vi "State Machine Kernel.vi"(4 "Init?":bool, 5 "Inputs":T3 {"Kobuki Sensors"."Charger Source" items=["DISCHARGING"=0, "DOCKING_CHARGED"=2, "DOCKING_CHARGING"=6, "ADAPTER_CHARGED"=18, "ADAPTER_CHARGING"=22]; "accelerometer"."z axis (g)" format="%.3f"; "accelerometer"."y axis (g)" format="%.3f"; "accelerometer"."x axis (g)" format="%.3f"}, 7 "StateIn":T1=enum."Init") -> (0 "Terminated?":bool, 2 "Outputs":T2, 3 "StateOut":T1=enum."Init")   [LabVIEW 2017]
uses:
  Statechart.lvsc/Inputs.ctl
  shared/Accelerometer.ctl
  Kobuki/KobukiSensors.ctl
  Kobuki/Kobuki Bumps and WheelDrops.ctl
  Kobuki/Kobuki Buttons.ctl
  Statechart.lvsc/Outputs.ctl
  StatesEnum.ctl
  Statechart.lvsc
panel:
  # "Electrical: charging, battery, OI mode"
  # "Sensors: bump, cliff, button, wheel drop"
  # "Motors:"
  # "Inertia"
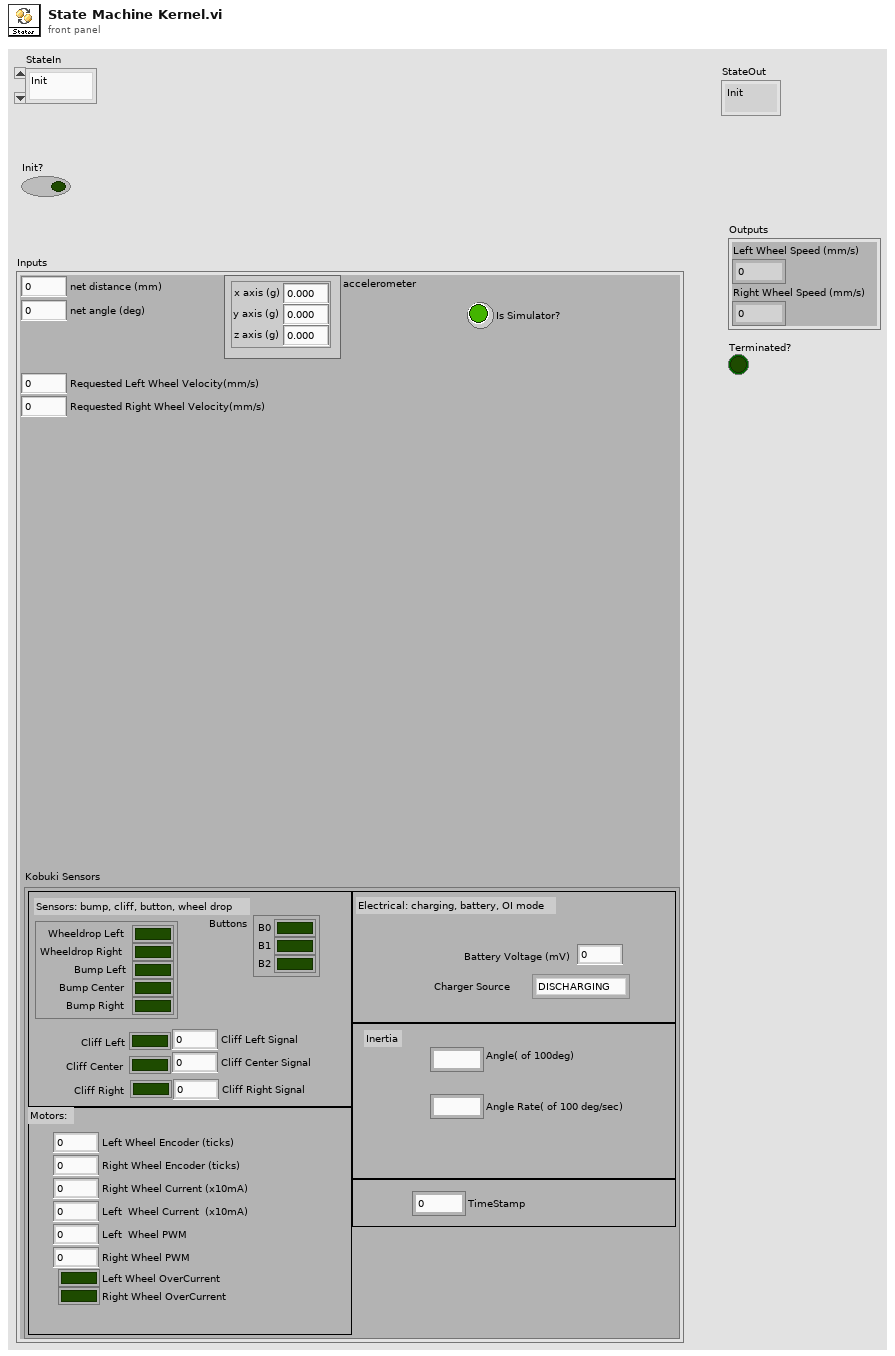
[diagram p1: front panel]
types:
  T1 = typedef "StatesEnum.ctl" = enum16{"Pause", "Init", "Shut"}
  T2 = typedef "Statechart.lvsc/Outputs.ctl" = cluster{"Left Wheel Speed (mm/s)":i16, "Right Wheel Speed (mm/s)":i16}
  T3 = typedef "Statechart.lvsc/Inputs.ctl" = cluster{"net distance (mm)":i32, "net angle (deg)":i32, "accelerometer":T4, "Is Simulator?":bool, "Kobuki Sensors":T5, "Requested Left Wheel Velocity(mm/s)":i32, "Requested Right Wheel Velocity(mm/s)":i32}
  T4 = typedef "Accelerometer.ctl" = cluster{"x axis (g)":dbl, "y axis (g)":dbl, "z axis (g)":dbl}
  T5 = typedef "KobukiSensors.ctl" = cluster{"Bumps + Wheel Drops":T6, "Cliff Left":bool, "Cliff Center":bool, "Cliff Right":bool, "Cliff Left Signal":u16, "Cliff Center Signal":u16, "Cliff Right Signal":u16, "Buttons":T7, "Left Wheel Encoder (ticks)":u16, "Right Wheel Encoder (ticks) ":u16, "Left  Wheel PWM":i8, "Right Wheel PWM":i8, "Left Wheel OverCurrent":bool, "Right Wheel OverCurrent ":bool, "Right Wheel Current (x10mA)":i16, "Left  Wheel Current  (x10mA)":i16, "TimeStamp":u16, "Battery Voltage (mV)":i16, "Angle( of 100deg)":i16, "Angle Rate( of 100 deg/sec)":i16, "Charger Source ":i8}
  T6 = typedef "Kobuki Bumps and WheelDrops.ctl" = cluster{"Wheeldrop Left":bool, "Wheeldrop Right":bool, "Bump Left":bool, "Bump Center":bool, "Bump Right":bool}
  T7 = typedef "Kobuki Buttons.ctl" = cluster{"B0":bool, "B1":bool, "B2":bool}
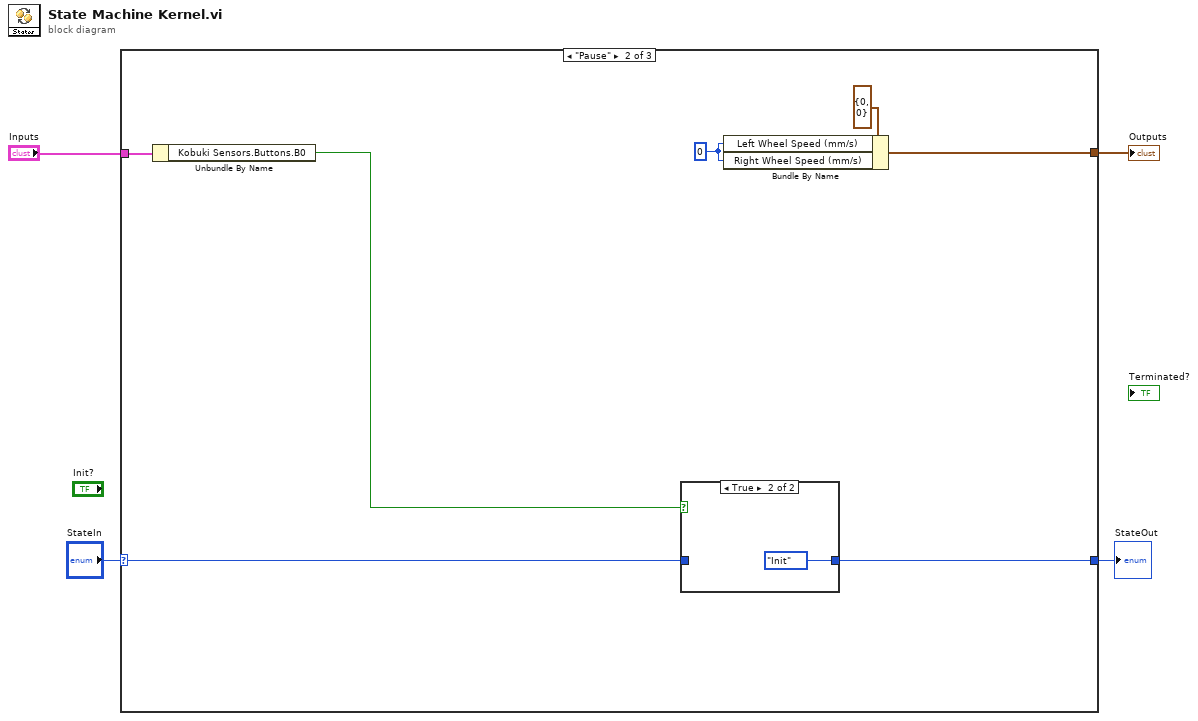
[diagram p0: block diagram]
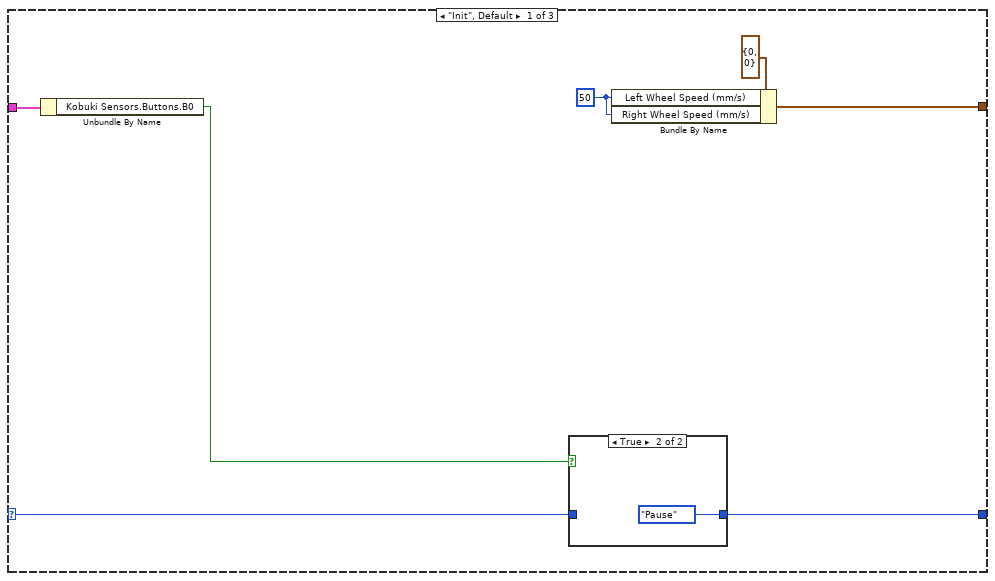
[diagram p2: hidden frame]
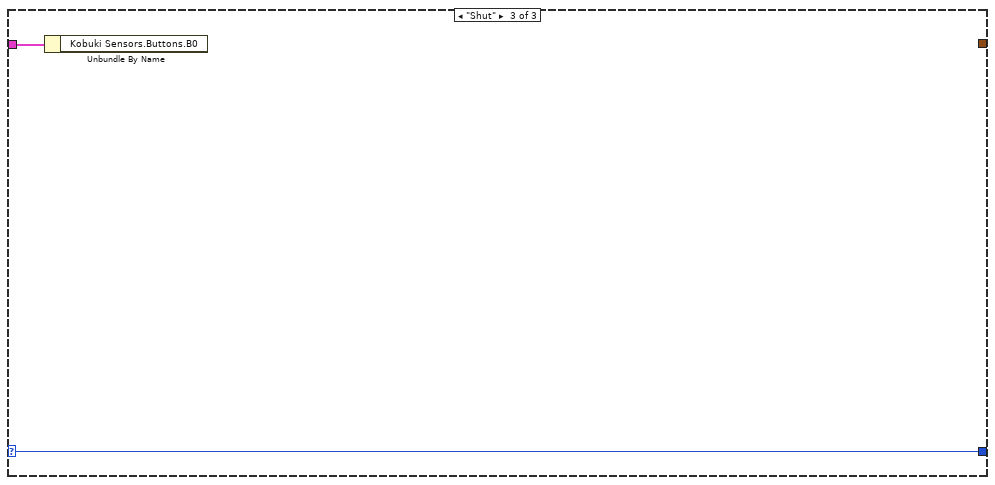
[diagram p5: hidden frame]
diagram:
  n1 = case shown="\"Pause\"" "StateIn" {
    selector: "StateIn" -> [w6 w15 w24]
    tunnel: [w5 w14 w24] -> w3
    tunnel: "Inputs" -> [w7 w16 w23]
    tunnel: [w11 w20 _] -> w2
    frame "Init", Default {
      w9 = i16 50 ("Left Wheel Speed (mm/s)")
      n2 = Unbundle By Name(w7) -> ("Kobuki Sensors.Buttons.B0"=w8:bool)
      n3 = case shown="True" w8 {
        tunnel: w6 -> [w12 _]
        tunnel: [w12 StatesEnum."Pause" ("StateIn")] -> w5
        frame False {
        }
        frame True {
        }
      }
      n4 = Bundle By Name(cluster=T2 {"Left Wheel Speed (mm/s)"=0, "Right Wheel Speed (mm/s)"=0} ("Outputs 2"), "Left Wheel Speed (mm/s)"=w9, "Right Wheel Speed (mm/s)"=w9) -> (w11:T2)
    }
    frame "Pause" {
      w18 = i16 0 ("Left Wheel Speed (mm/s)")
      n5 = Unbundle By Name(w16) -> ("Kobuki Sensors.Buttons.B0"=w17:bool)
      n6 = case shown="True" w17 {
        tunnel: w15 -> [w21 _]
        tunnel: [w21 StatesEnum."Init" ("StateIn")] -> w14
        frame False {
        }
        frame True {
        }
      }
      n7 = Bundle By Name(cluster=T2 {"Left Wheel Speed (mm/s)"=0, "Right Wheel Speed (mm/s)"=0} ("Outputs 2"), "Left Wheel Speed (mm/s)"=w18, "Right Wheel Speed (mm/s)"=w18) -> (w20:T2)
    }
    frame "Shut" {
      n8 = Unbundle By Name(w23) -> ()  [unwired: 1 out]
    }
  }
  "Outputs" <- w2
  "StateOut" <- w3
